vi "RewindButton_Create.vi"(0 "reference in":refnum<class "RewindButton.lvclass">, 11 "Error In":errorcluster) -> (4 "reference out":refnum<class "RewindButton.lvclass">, 15 "Error Out":errorcluster)   [LabVIEW 2024, in "RewindButton.lvclass"]
uses:
  RewindButton.lvclass/RewindButton.ctl
  RewindButton.lvclass
  C:/Users/burakkorkmaz/Desktop/Leveling/labview-desing-patterns/Command Pattern/Client/Buttons/Button_class/Button.lvclass
  C:/Users/burakkorkmaz/Desktop/Leveling/labview-desing-patterns/Command Pattern/Client/Buttons/RewindButton_class/RewindButton.lvclass
  Button_class/Button.lvclass
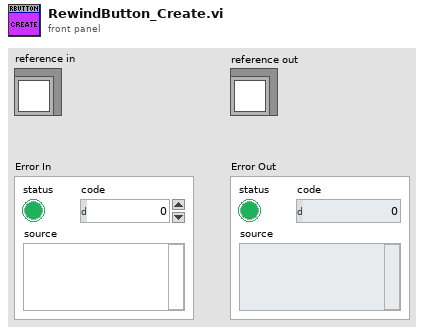
[diagram p1: front panel]
types:
  T1 = typedef "G4SubTemplate_Simple_5x6x5.lvclass/ObjectAttributes.ctl" = cluster{"Attribute1":dbl}
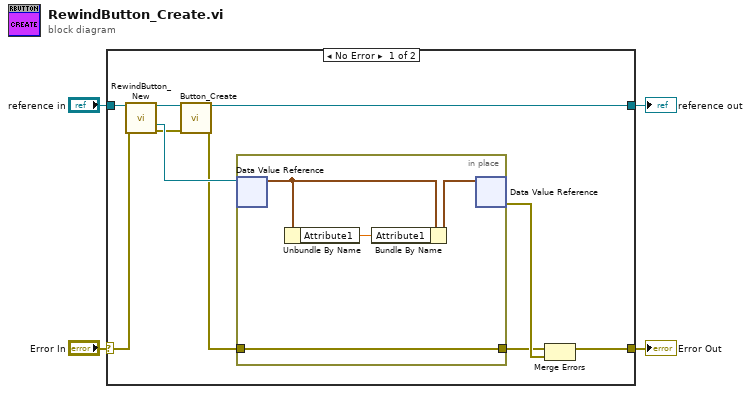
[diagram p0: block diagram]
diagram:
  n1 = case shown="No Error" "Error In" {
    selector: "Error In" -> [w10 w20]
    tunnel: [w8 w20] -> w3
    tunnel: "reference in" -> [w12 w19]
    tunnel: [w7 w19] -> w1
    frame No Error {
      n2 = call "RewindButton_New.vi"("reference in"=w12, "Error In"=w10) -> ("reference out"=w13:refnum<class "RewindButton.lvclass">, "DVRRefOut"=w14:refnum<data-value>, "Error Out"=w11:errorcluster)  [unwired: 10 in, 1 out]
      n3 = call "Button_Create.vi"("reference in"=w13, "Error In"=w11) -> ("reference out"=w7:refnum<class "RewindButton.lvclass">, "Error Out"=w6:errorcluster)  [unwired: 12 in]
      n4 = in-place {
        in-place-border: w6 -> [w15]
        in-place-border: [w15] -> w5
        n5 = in-place-dvr #1(w14) -> (w17:T1)  [unwired: 1 out]
        n6 = Unbundle By Name(w17) -> ("Attribute1"=w16:dbl)
        n7 = Bundle By Name(cluster=w17, "Attribute1"=w16) -> (w18:T1)
        n8 = in-place-dvr #1(w18) -> (w9:errorcluster)  [unwired: 1 out]
      }
      n9 = Merge Errors(w5, w9) -> (w8:errorcluster)
    }
    frame Error {
    }
  }
  "Error Out" <- w3
  "reference out" <- w1
